vi "Configure Measurement.vi"(6 "Manual Range (1.0)":dbl=1.0, 7 "Absolute Resolution (0.01)":dbl=0.01, 8 "error in (no error)":errorcluster, 9 "Auto Range (T:Enable)":bool=TRUE, 10 "Function (0: DC Volts)":u16(ring) items=["DC Volts", "AC Volts", "DC Current", "AC Current", "2-Wire Resistance", "4-Wire Resistance"], 11 "VISA resource name":refnum<visa-resource-name>) -> (0 "error out":errorcluster, 3 "VISA resource name out":refnum<visa-resource-name>)   [LabVIEW 2024, in "EFmeter.lvlib"]
doc: "Configures the measurement type, resolution, and range on the instrument."
uses:
  <instrlib>/EFmeter/EFmeter.lvlib
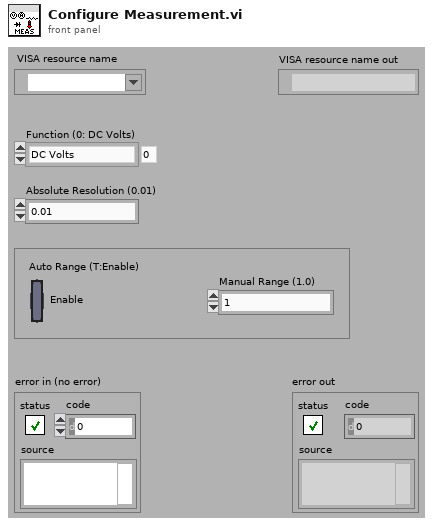
[diagram p1: front panel]
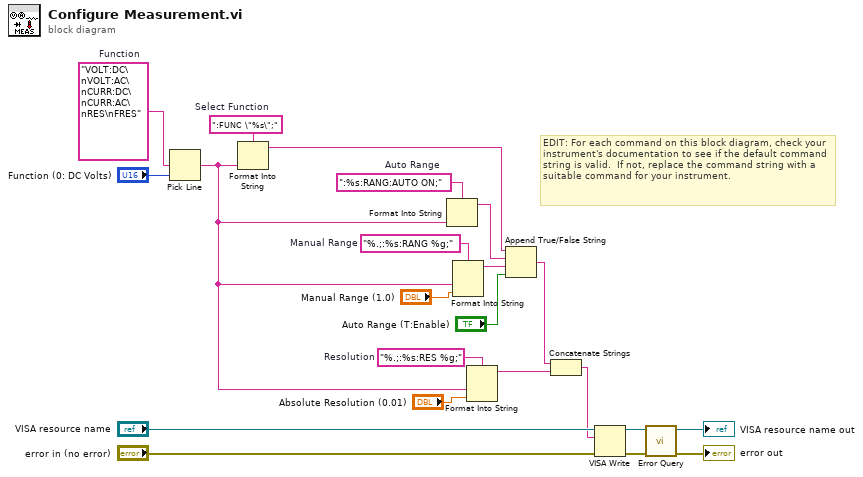
[diagram p0: block diagram]
diagram:
  w10 = ":%s:RANG:AUTO ON;"  # Auto Range
  w12 = "%.;:%s:RANG %g;"  # Manual Range
  w15 = "%.;:%s:RES %g;"  # Resolution
  w16 = ":FUNC \"%s\";"  # Select Function
  w18 = "VOLT:DC\nVOLT:AC\nCURR:DC\nCURR:AC\nRES\nFRES"  # Function
  # "EDIT: For each command on this block diagram, check your instrument's documentation to see if the default command string is valid.  If not, replace the command string with a suitable command for your instrument."
  n1 = Pick Line(multi-line string=w18, line index="Function (0: DC Volts)") -> (output string=w6:string)  [unwired: 1 in]
  n2 = Format Into String(format string=w16, w6) -> (resulting string=w4:string)  [unwired: 2 in, 1 out]
  n3 = Format Into String(format string=w10, w6) -> (resulting string=w9:string)  [unwired: 2 in, 1 out]
  n4 = Format Into String(format string=w12, w6, "Manual Range (1.0)") -> (resulting string=w11:string)  [unwired: 2 in, 1 out]
  n5 = Format Into String(format string=w15, w6, "Absolute Resolution (0.01)") -> (resulting string=w2:string)  [unwired: 2 in, 1 out]
  n6 = Append True/False String(1:"Auto Range (T:Enable)", 2:w11, 3:w9, 4:w4) -> (0:w3:string)
  n7 = Concatenate Strings(w3, w2) -> (w1:string)
  n8 = VISA Write(VISA resource name="VISA resource name", write buffer=w1, error in (no error)="error in (no error)") -> (VISA resource name out=w14:refnum<visa-resource-name>, error out=w13:errorcluster)  [unwired: 1 out]
  n9 = call <instrlib>:"Error Query.vi"("error in (no error)"=w13, "VISA resource name"=w14) -> ("error out"=→"error out":errorcluster, "VISA resource name out"=→"VISA resource name out":refnum<visa-resource-name>)  [unwired: 6 in, 2 out]
